vi "Configure Marker Frequency Counter.vi"(8 "error in (no error)":errorcluster {"code" format="%.0x"}, 9 "frequency counter resolution":dbl, 10 "marker frequency counter (Off)":bool, 11 "instrument handle":refnum<k15>) -> (0 "error out":errorcluster {"code" format="%.0x"}, 3 "instrument handle out":refnum<k15>)   [LabVIEW 2009, in "Keysight XSAn.lvlib"]
doc: "This function sets the marker frequency counter resolution and turns the marker frequency counter on/off.\n\nSupported Models:M9290A, N8973B, N8974B, N8975B, N8976B, N9000A, N9000B, N9010A, N9010B, N9020A, N9020B, N9030A, N9030B, N9038A, N9040B, N9041B, SPN9003A, SPN9026A"
uses:
  <instrlib>/Keysight XSAn/Keysight XSAn.lvlib
  AgXSAn.dll
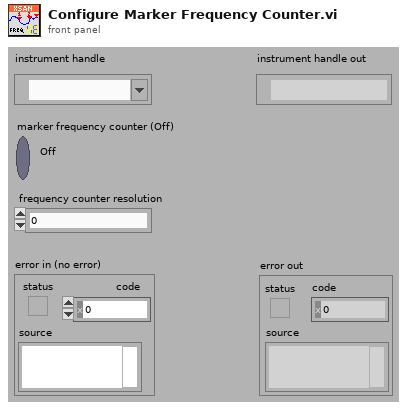
[diagram p1: front panel]
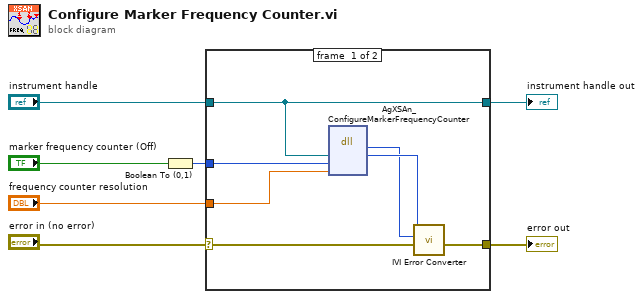
[diagram p0: block diagram]
diagram:
  n1 = Boolean To (0,1)(Boolean="marker frequency counter (Off)") -> (0, 1=w1:i16)
  n2 = case shown="No Error" "error in (no error)" {
    selector: "error in (no error)" -> [w12 w16]
    tunnel: [w13 w16] -> w6
    tunnel: "instrument handle" -> [w9 w15]
    tunnel: [w9 w15] -> w4
    tunnel: "frequency counter resolution" -> [w10 _]
    tunnel: w1 -> [w8 _]
    frame #0 {
      n3 = dll-call lib="AgXSAn**.dll" fn="AgXSAn_ConfigureMarkerFrequencyCounter" ("LabVIEW:IviSpecAn_ConfigureMarkerFrequencyCounter")("instrument handle"=w9, "marker frequency counter"=w8, "frequency counter resolution"=w10) -> ("Status"=w11:i32, "instrument handle"=w14:u32)  [unwired: 5 in, 2 out]
      n4 = call <instrlib>:"IVI Error Converter.vi"("error in (no error)"=w12, "IVI error code (0)"=w11, "instrument handle"=w14) -> ("error out"=w13:errorcluster)  [unwired: 7 in, 1 out]
    }
    frame #1 {
    }
  }
  "error out" <- w6
  "instrument handle out" <- w4
